vi "add point.vi"(7 "coordinates":T2, 9 "Point information":T1={"Time UTC"="", "Heading"="", "Name path/point"="<Placemark>", "description"=""}, 10 "string KLM in":string) -> (3 "string KLM out":string)   [LabVIEW 2015, in "Biblioteka moduł map v3.lvlib" / "KML.lvlib"]
uses:
  KML.lvlib
  KML point information.ctl
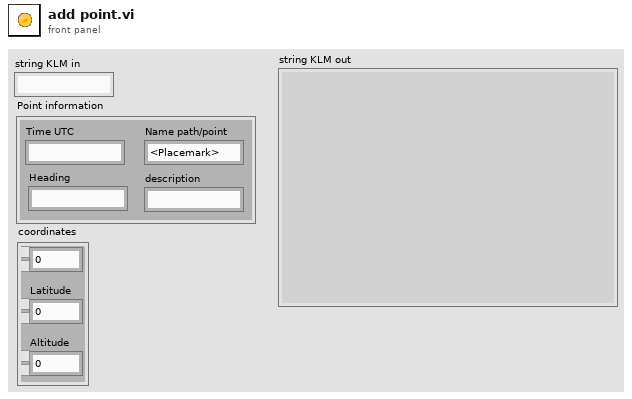
[diagram p1: front panel]
types:
  T1 = typedef "Biblioteka moduł map v3.lvlib/KML.lvlib/KML point information.ctl" = cluster{"Time UTC":string, "Heading":string, "Name path/point":string, "description":string}
  T2 = cluster{"Longitude":dbl, "Latitude":dbl, "Altitude":dbl}
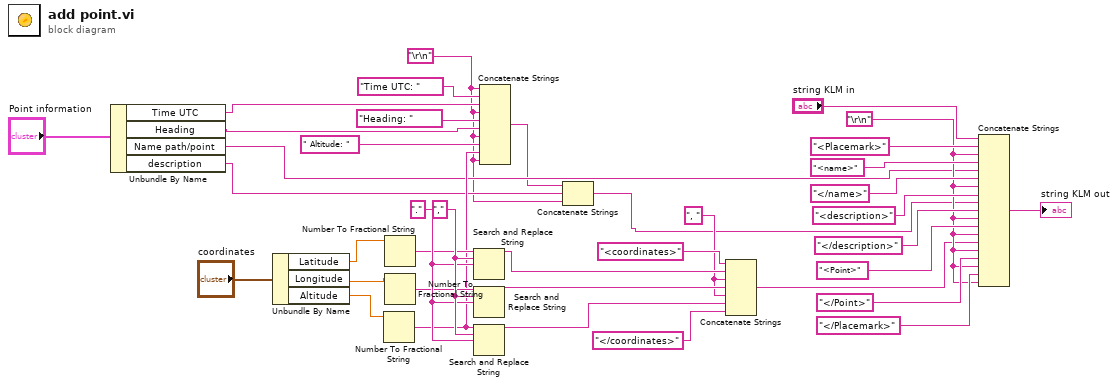
[diagram p0: block diagram]
diagram:
  w2 = "\r\n"
  w20 = ", " ("string")
  w30 = "." ("search string")
  w31 = "," ("search string")
  w26 = "\r\n"
  n1 = Unbundle By Name("Point information") -> ("Time UTC"=w7:string, "Heading"=w6:string, "Name path/point"=w5:string, "description"=w4:string)
  n2 = Unbundle By Name("coordinates") -> ("Latitude"=w15:dbl, "Longitude"=w14:dbl, "Altitude"=w13:dbl)
  n3 = Number To Fractional String(number=w13) -> (F-format string=w9:string)  [unwired: 3 in]
  n4 = Number To Fractional String(number=w15) -> (F-format string=w16:string)  [unwired: 3 in]
  n5 = Number To Fractional String(number=w14) -> (F-format string=w17:string)  [unwired: 3 in]
  n6 = Search and Replace String(input string=w16, search string=w31, replace string=w30) -> (result string=w22:string)  [unwired: 5 in, 3 out]
  n7 = Search and Replace String(input string=w17, search string=w31, replace string=w30) -> (result string=w21:string)  [unwired: 5 in, 3 out]
  n8 = Search and Replace String(input string=w9, search string=w31, replace string=w30) -> (result string=w19:string)  [unwired: 5 in, 3 out]
  n9 = Concatenate Strings(w2, "Time UTC: " ("search string"), w7, w2, "Heading: " ("search string"), w6, w2, " Altitude: " ("Altitude:"), w9, w2) -> (w1:string)
  n10 = Concatenate Strings(w1, w4, w2) -> (w3:string)
  n11 = Concatenate Strings("<coordinates>" ("string"), w22, w20, w21, w20, w19, "</coordinates>" ("string")) -> (w23:string)
  n12 = Concatenate Strings("string KLM in", "<Placemark>", w26, "<name>", w5, "</name>", w26, "<description>", w3, "</description>", w26, "<Point>", w26, w23, w26, "</Point>", w26, "</Placemark>", w26) -> (→"string KLM out":string)
